vi "Load Get Icon Editor Context into memory.vi"   [LabVIEW 2021]
doc: "Loads Get Icon Editor Contex.vi relative to this VIs path.\n\nRelative Path: <projectfolder>\\resource\\plugins\\NIIconEditor\\Miscellaneous\\Icon Editor\\Get Icon Editor Context.vi\n\nThis is done to fix differences in the loading environment before calling Force Icon Editor To Unload.vi"
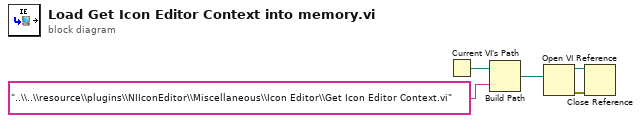
[diagram p0: block diagram]
diagram:
  n1 = Current VI's Path() -> (path=w4:path)
  n2 = Build Path(base path=w4, name or relative path="..\\..\\resource\\plugins\\NIIconEditor\\Miscellaneous\\Icon Editor\\Get Icon Editor Context.vi") -> (appended path=w3:path)
  n3 = Open VI Reference(vi path=w3) -> (vi reference=w1:refnum<vi>, error out=w2:errorcluster)  [unwired: 5 in]
  n4 = Close Reference(reference=w1, error in (no error)=w2) -> ()  [unwired: 1 out]
